vi "CAN_Send Diag Message.vi"(0 "Write Session in":refnum<k21>, 1 "Read Session in":refnum<k21>, 2 "Parttype ref":refnum<vi>, 3 "ODX File Path":path=path "C:/LegacyApp/DB_0CA_7100_4M0_0004_73710BVW3710/DB_0CA_7100_4M0_0004_73710BVW3710/DB_0CA_7100_4M0_0004_73710BVW3710.odx", 4 "Tx Msg":u8[](array[numeric])=[2, 26, 156, 255, 255, 255, 255, 255] format="%02x", 5 "error in (no error)":errorcluster, 6 "Enum":T2=enum."Get Calibration Status", 7 "Download CAL Progress":refnum<vi>, 10 "Postion":u16=3, 11 "Download CAL Time":refnum<vi>, 12 "Autotest":bool, 14 "ECU Info in":T1, 17 "Tester":refnum<k21>) -> (13 "Response Good?":bool, 15 "ECU Info":T1, 16 "pass?":bool, 18 "TxRx Data":string[][](array[string]), 19 "error out":errorcluster)   [LabVIEW 2018]
uses:
  Diagnostic Message.ctl
  typedefs/parttype.ctl
  <vilib>/xnet/xnet.llb/XNET Frame CAN.ctl
  <vilib>/xnet/xnet.llb/XNET Frame Type CAN.ctl
  CAN Communication VI's/Typedefs/Select Session.ctl
  typedefs/All Motions.ctl
  <vilib>/xnet/xnet.llb/XNET Write (Frame CAN).vi
  <vilib>/xnet/xnet.llb/XNET Read (Frame CAN).vi
panel:
  out "Error String Out 2":string
  out "pass?_FBL":bool
  out "Rx Message":u8[](array[numeric]) format="%02x"
  out "Error String Out":string
  in  "Tx Arbitration Id":u32=402391172 format="%.0x"
  out "Part Number":string
  out "Vehicle Type":string
  out "SW level":string
  out "Calibrated":bool
  out "HW level":string
  out "CAL level":string
  out "Boot level":string
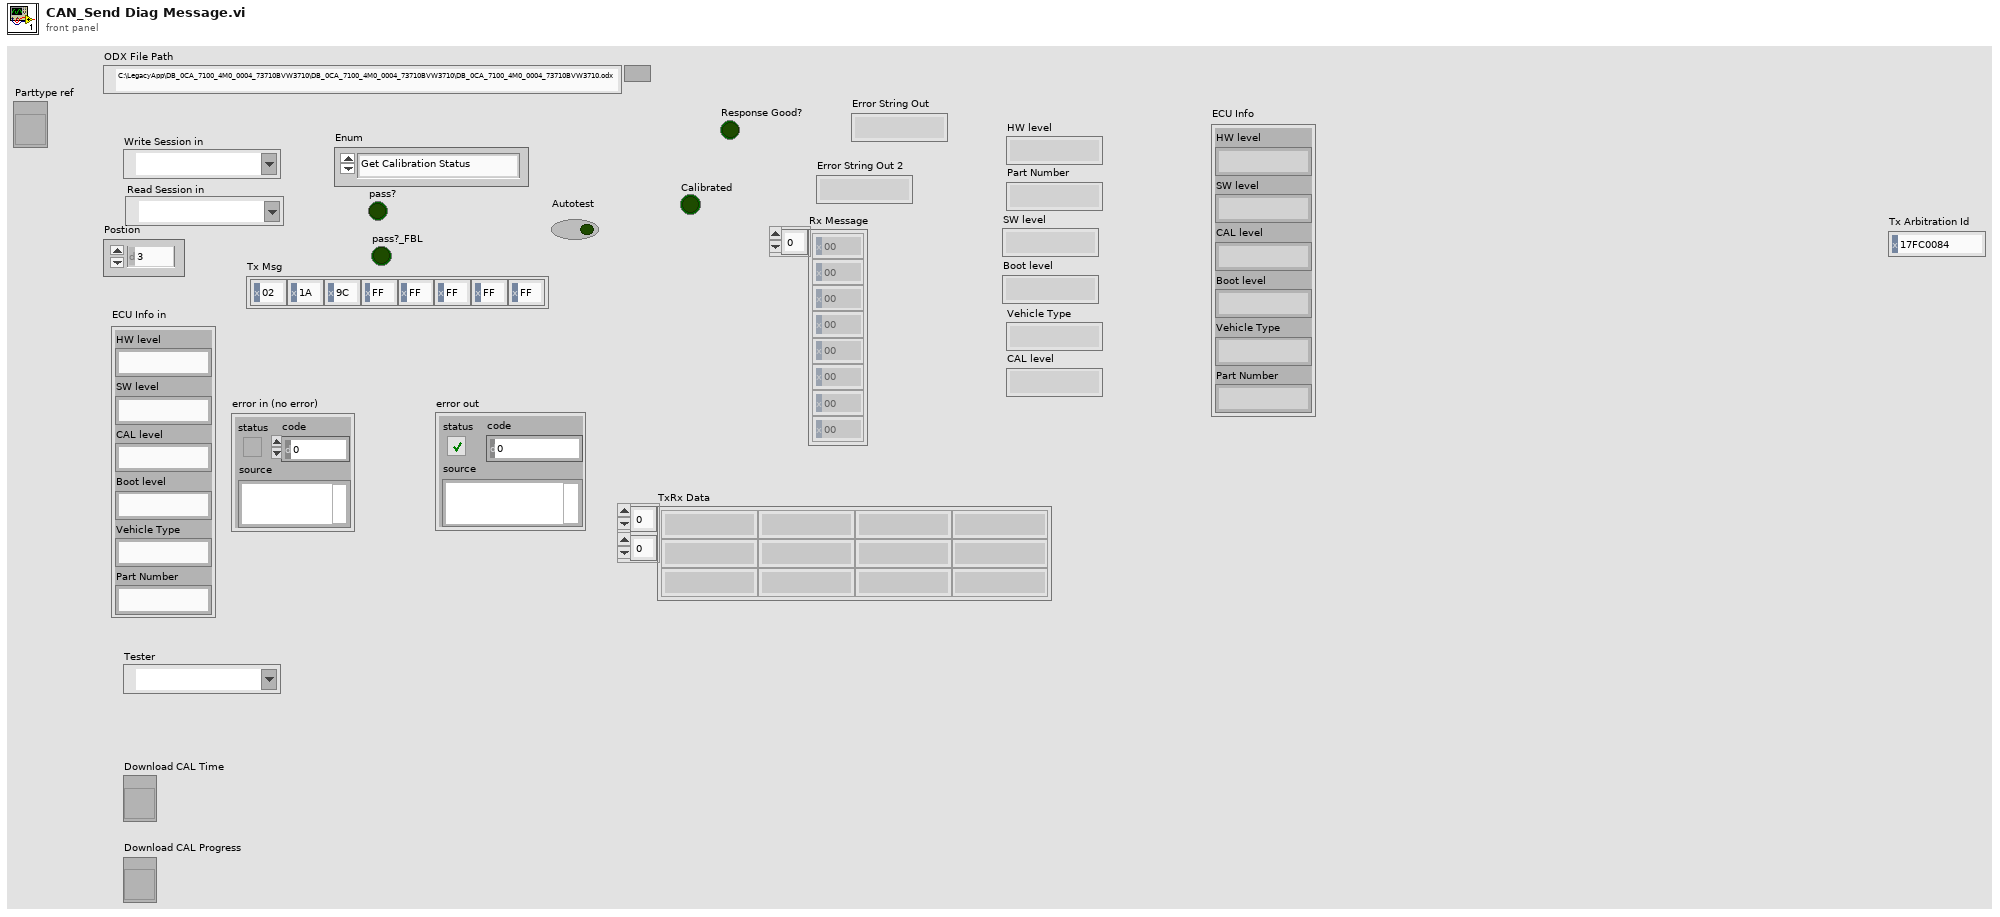
[diagram p1: front panel]
types:
  T1 = cluster{"HW level":string, "SW level":string, "CAL level":string, "Boot level":string, "Vehicle Type":string, "Part Number":string}
  T2 = typedef "Diagnostic Message.ctl" = enum16{"User Select", "Get User Multi-Frame", "Diag Session Prog", "Diag Session Ext", "Diag Session EOL", "Diag Session Default", "Diag Session Dev", "Read Active Session", "Read HW", "Read SW", "Read Part Number", "Learn Start Glass", "Learn Start Rollo", "Get Calibration Status", "Read SW CAL Boot", "Go to Position", "Get Parametric Mode Status", "Enable Parametric Mode", "Disable Parametric Mode", "Enable Production Mode", "Disable Production Mode", "Reset ECU", "Go to Slide Close", "Go to Slide Open", "Go to Vent Open", "Rollo Open", "Rollo Close", "Write Vehicle Type", "Read Vehicle Type", "Clear DTC", "Check Teach DTC", "Write Shop Code", "Download CAL", "Finish Flash", "Delete RP RF", "Download FBL"}
  T3 = typedef "XNET Frame CAN.ctl" = cluster{"timestamp":timestamp, "payload":u8[], "identifier":u32, "type":T4, "extended?":bool, "echo?":bool}
  T4 = typedef "XNET Frame Type CAN.ctl" = u8
  T5 = typedef "Select Session.ctl" = enum16{"DefaultSession", "Development", "Extended", "EOL", "Programming"}
  T6 = typedef "All Motions.ctl" = enum16{"Idle", "Glass Teach", "Glass Slide Open", "Glass Slide Open 2", "Glass Slide Close", "Glass Slide Close 2", "Glass Vent Open", "Glass Vent Close", "Sunshade Teach", "Sunshade Teach 2", "Sunshade Open", "Sunshade Open 2", "Sunshade Close", "Sunshade Close 2", "Glass Slide Open Sunshade Open", "Glass Slide Open 2 Sunshade Open", "Glass Slide Open Sunshade Close", "Glass Slide Open 2 Sunshade Close", "Glass Slide Close Sunshade Open", "Glass Slide Close 2 Sunshade Open", "Glass Slide Close Sunshade Close", "Glass Slide Close 2 Sunshade Close", "Glass Vent Open Sunshade Open", "Glass Vent Open Sunshade Close", "Glass Vent Close Sunshade Open", "Glass Vent Close Sunshade Close", "Express Glass Slide Open", "Express Glass Slide Open 2", "Express Glass Slide Close", "Express Glass Slide Close 2", "Express Glass Vent Open", "Express Glass Vent Close", "Express Sunshade Open", "Express Sunshade Close", "Express Sunshade Open 2", "Express Sunshade Close 2", "Express Glass Slide Open Sunshade Open", "Express Glass Slide Open 2 Sunshade Open", "Express Glass Slide Open Sunshade Close", "Express Glass Slide Open 2 Sunshade Close", "Express Glass Slide Close Sunshade Open", "Express Glass Slide Close 2 Sunshade Open", "Express Glass Slide Close Sunshade Close", "Express Glass Slide Close 2 Sunshade Close", "Express Glass Vent Open Sunshade Open", "Express Glass Vent Open Sunshade Close", "Express Glass Vent Close Sunshade Open", "Express Glass Vent Close Sunshade Close", "Goto Position Glass", "Goto Position Sunshade"}
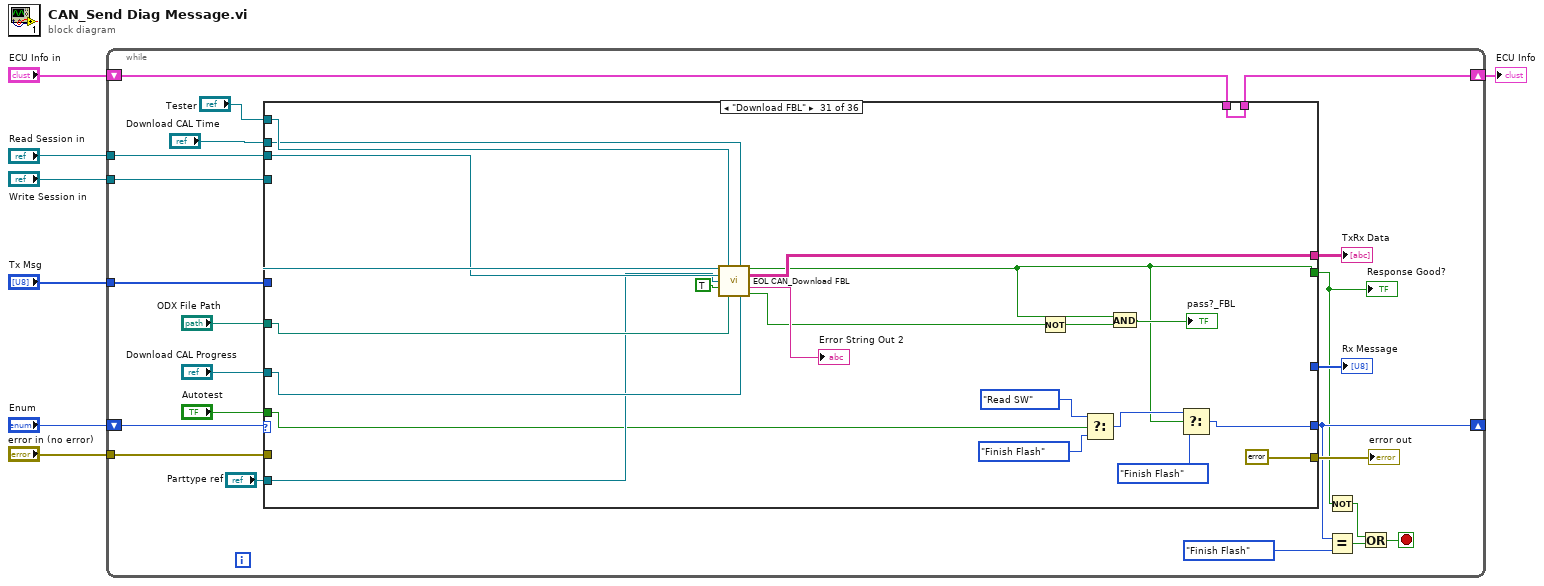
[diagram p0: block diagram]
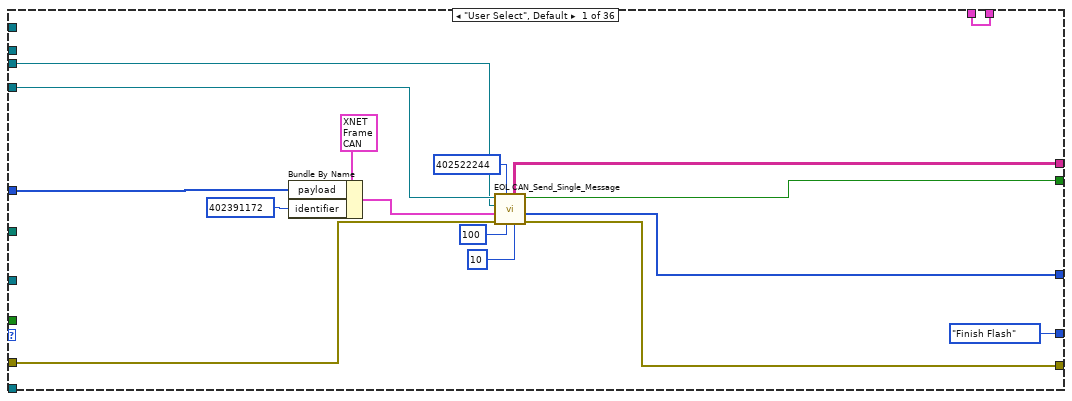
[diagram p2: hidden frame]
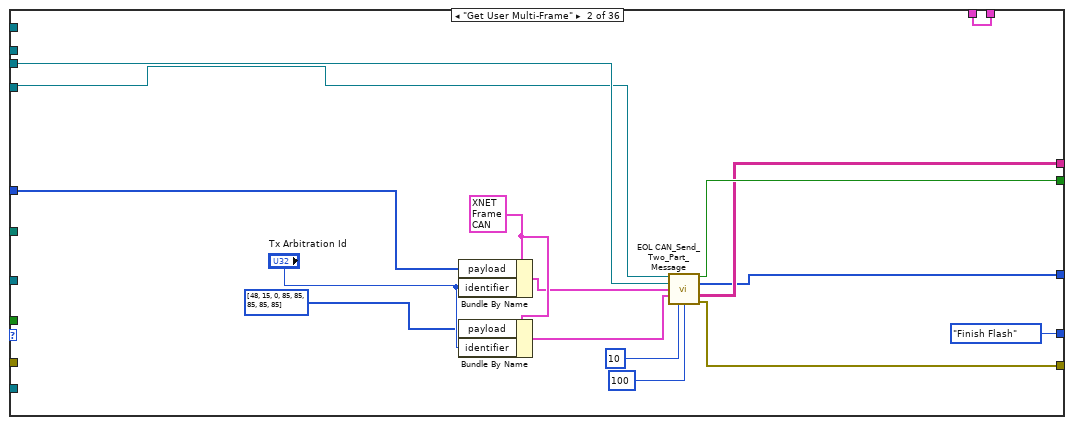
[diagram p3: hidden frame]
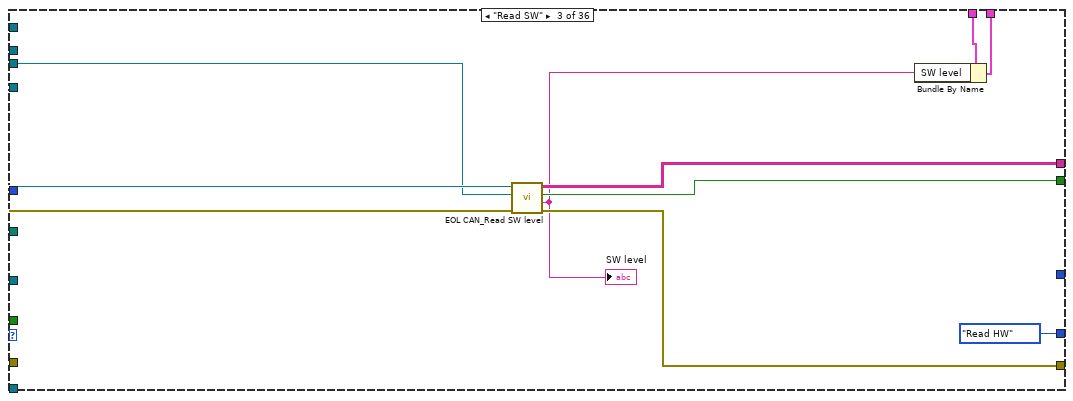
[diagram p4: hidden frame]
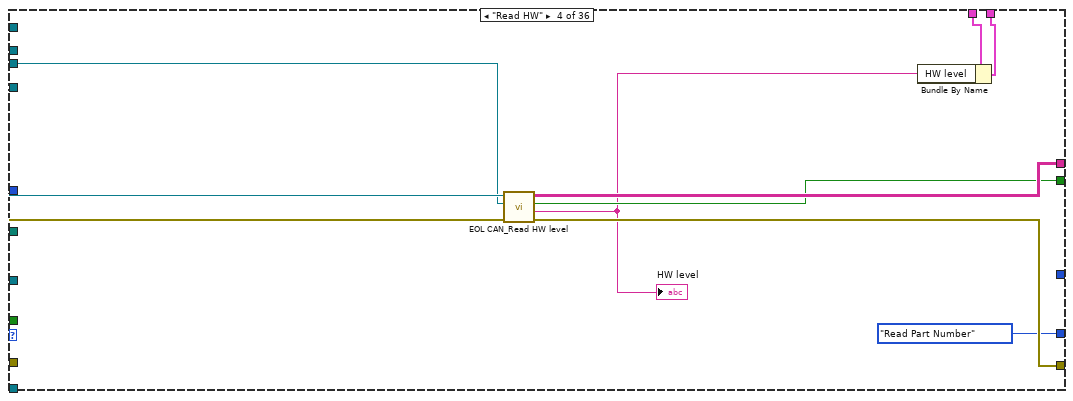
[diagram p5: hidden frame]
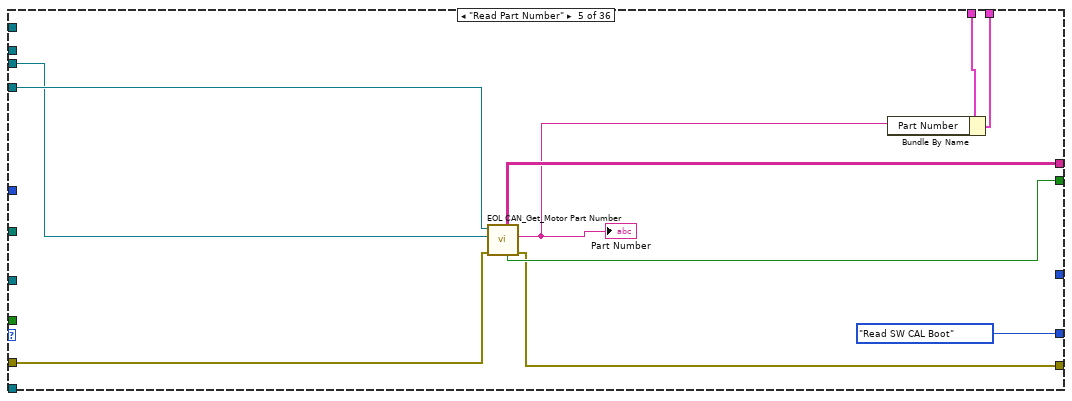
[diagram p6: hidden frame]
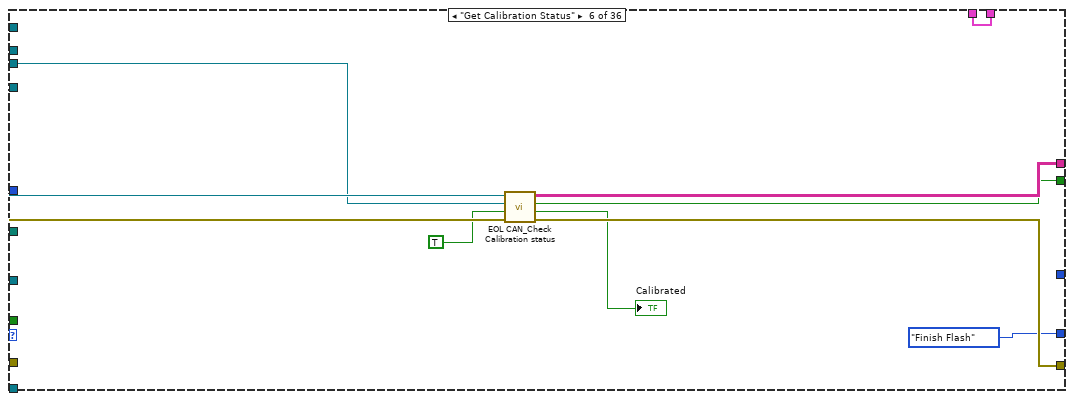
[diagram p7: hidden frame]
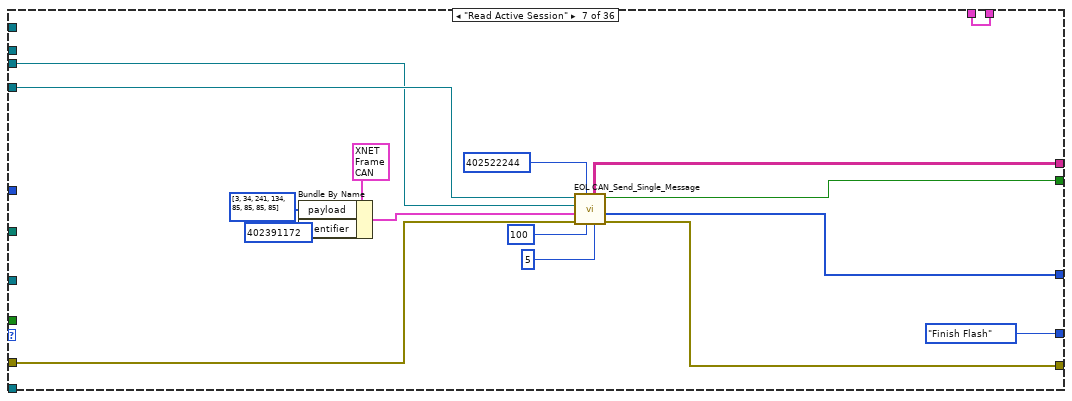
[diagram p8: hidden frame]
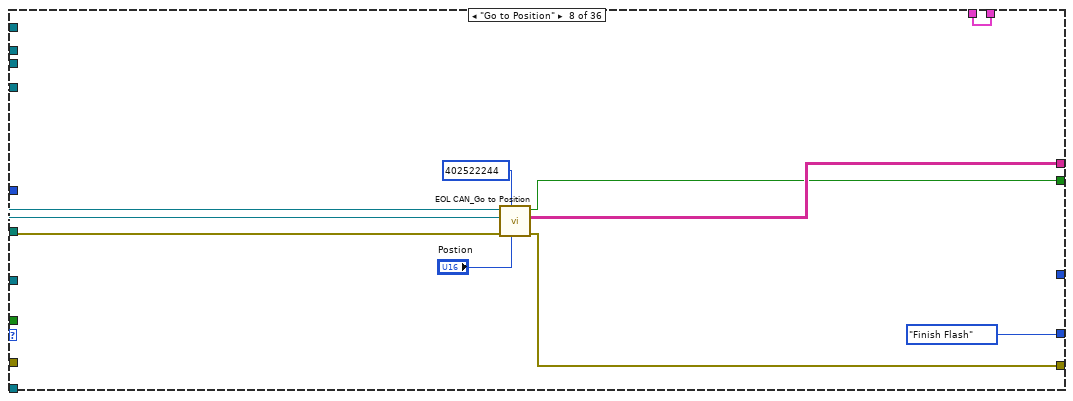
[diagram p9: hidden frame]
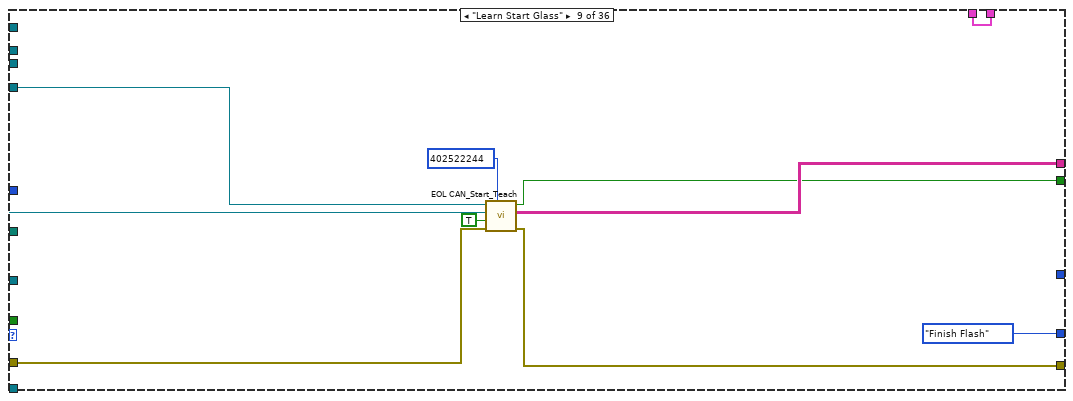
[diagram p10: hidden frame]
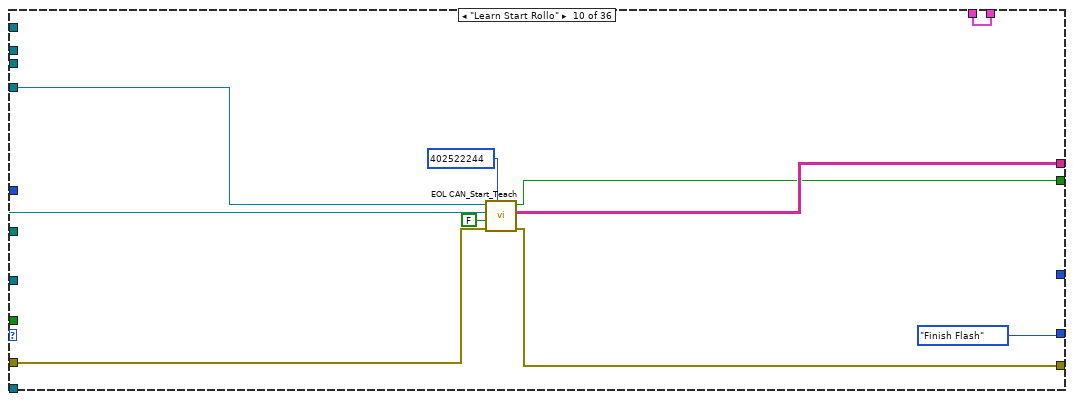
[diagram p11: hidden frame]
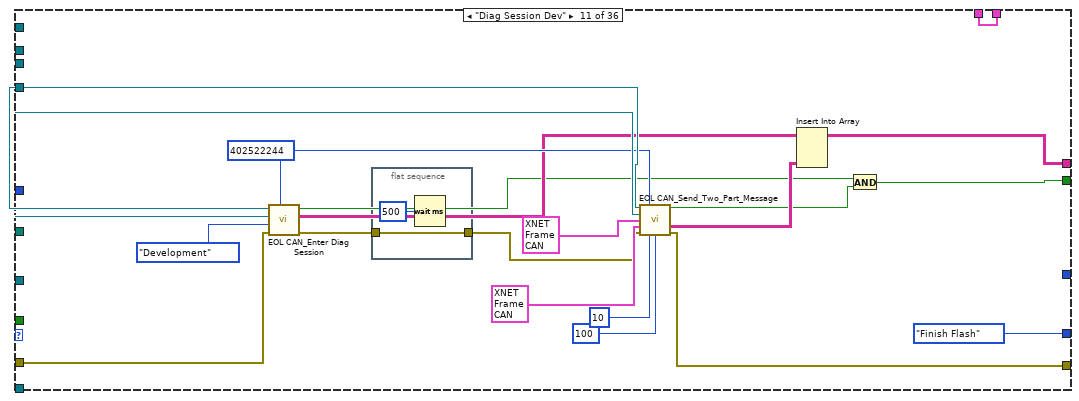
[diagram p12: hidden frame]
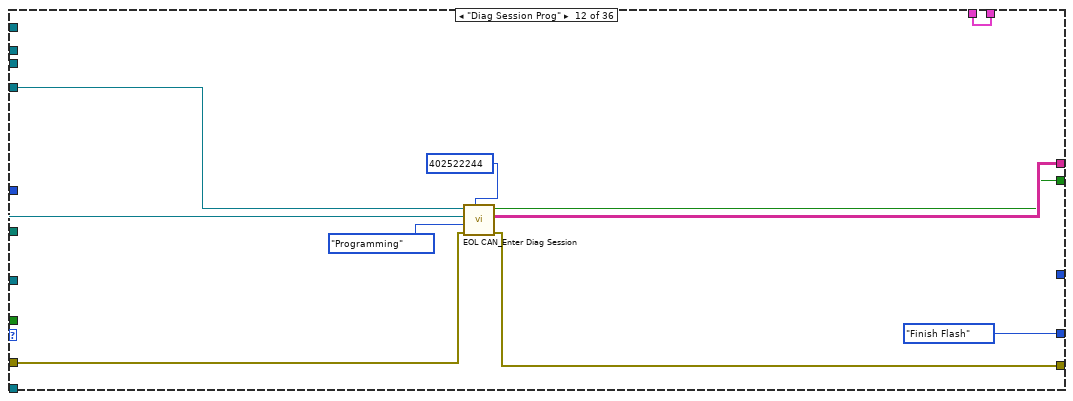
[diagram p13: hidden frame]
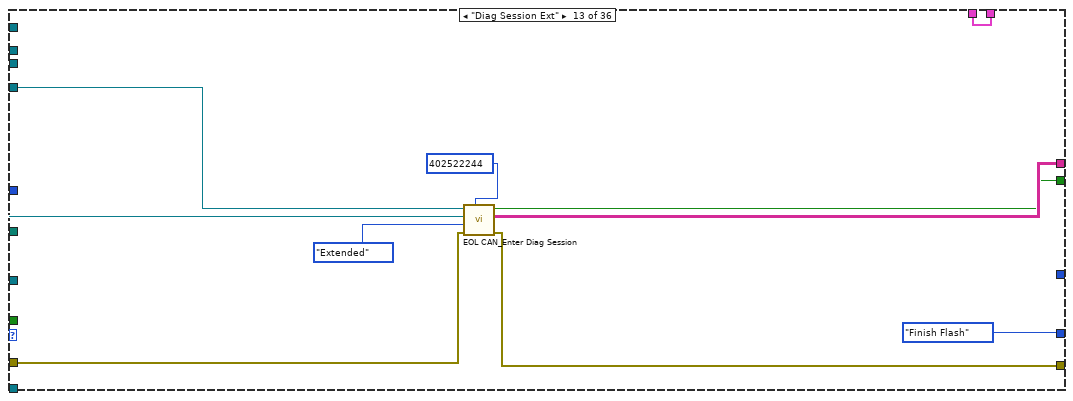
[diagram p14: hidden frame]
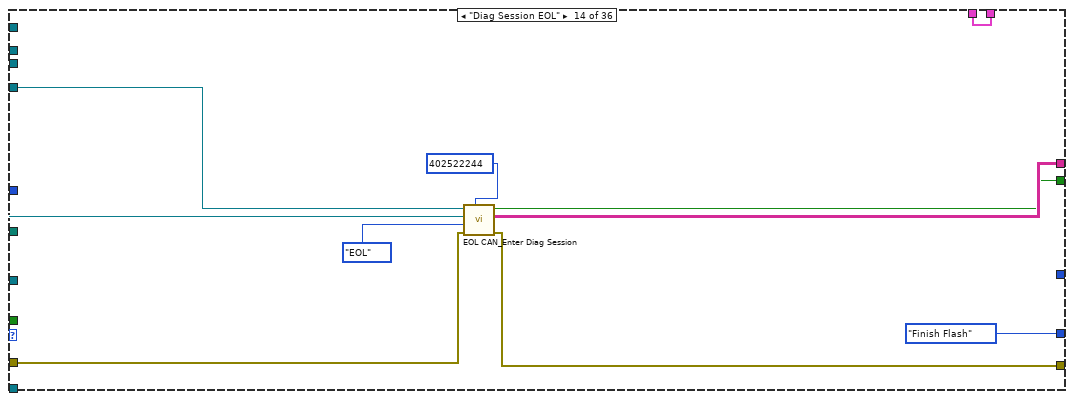
[diagram p15: hidden frame]
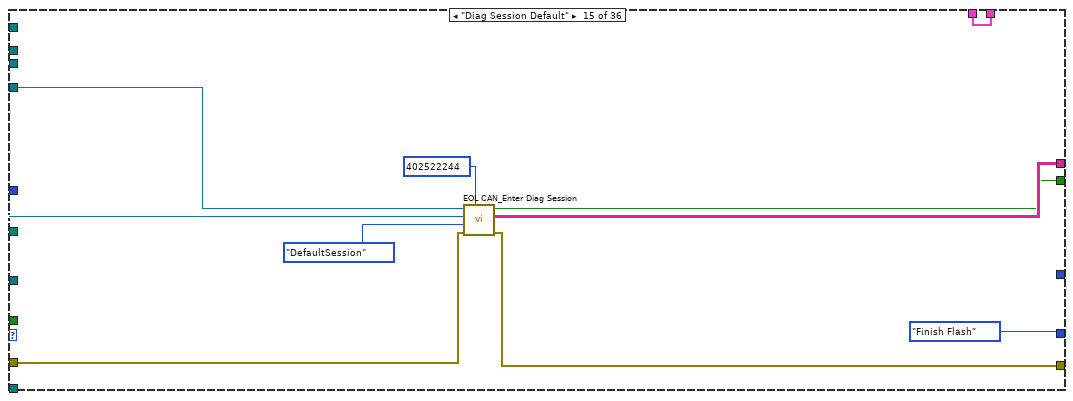
[diagram p16: hidden frame]
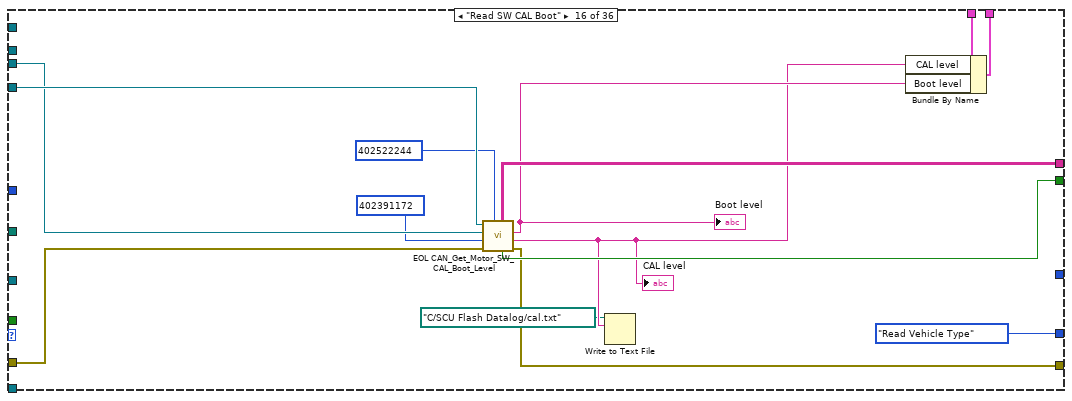
[diagram p17: hidden frame]
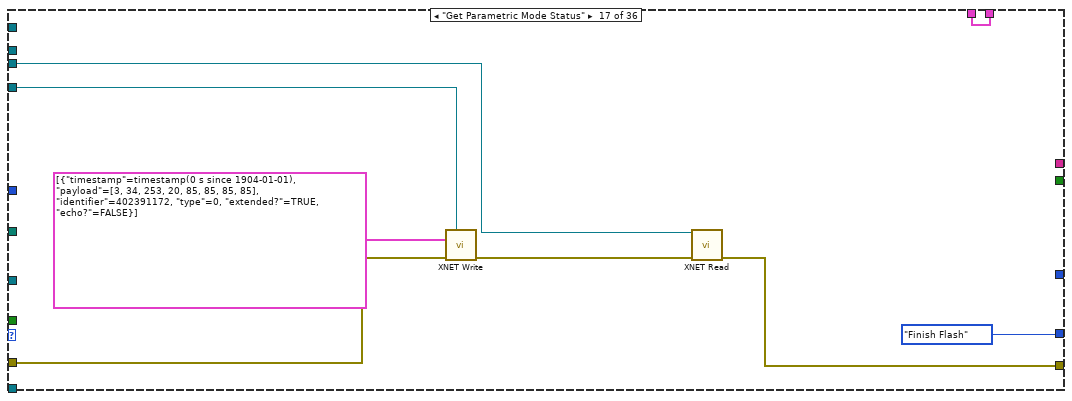
[diagram p18: hidden frame]
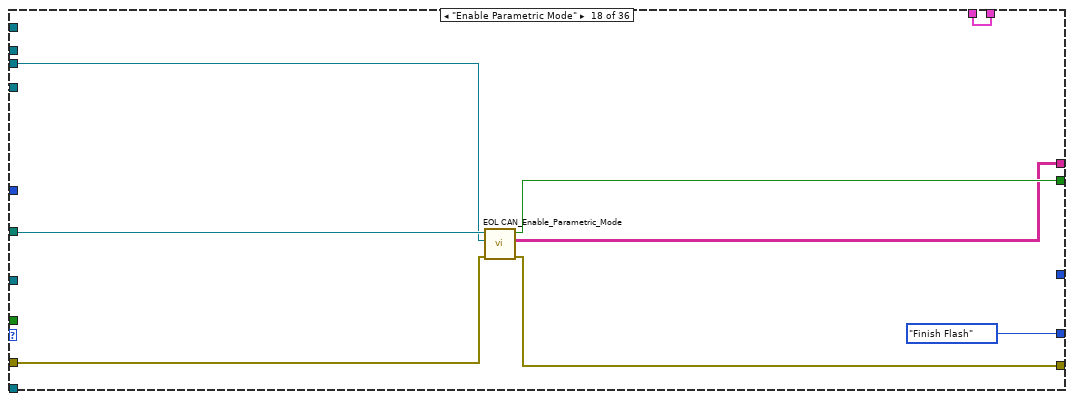
[diagram p19: hidden frame]
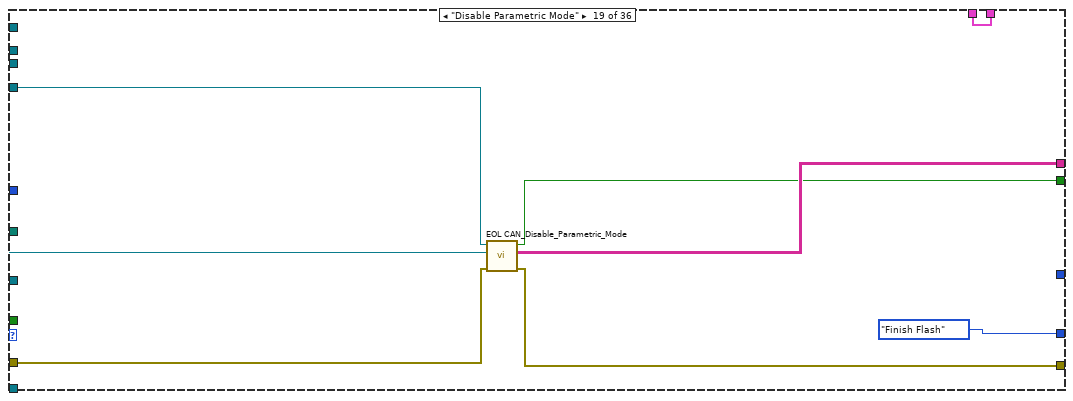
[diagram p20: hidden frame]
diagram:
  n1 = while {
    tunnel: "error in (no error)" -> [w29]
    tunnel: "Read Session in" -> [w27]
    tunnel: "Write Session in" -> [w26]
    shift-right: [w23] -> w3
    shift-left: "ECU Info in" -> [w22]
    tunnel: "Tx Msg" -> [w21]
    shift-right: [w16] -> _
    shift-left: "Enum" -> [w25]
    stop <- w19 stop-if-true
    n2 = case shown="\"Download FBL\"" w25 {
      tunnel: w27 -> [w44 w53 w66 w76 w89 w100 w116 w124 w135 w145 w163 w173 w183 w193 w203 w221 w229 w237 w242 w253 w261 w270 w280 w290 w300 w310 w320 w324 w332 w357 w379 w393 w400 w410 _ w439]
      tunnel: w26 -> [w45 w52 w67 w77 w90 w101 w117 w125 w136 w146 w165 w174 w184 w194 w204 w222 w231 w238 w243 w254 w262 w271 w281 w291 w301 w311 w321 w325 w333 w358 w380 w392 w401 w412 _ w440]
      tunnel: w29 -> [w43 _ w71 w81 w91 w99 w115 w127 w137 w147 w167 w179 w189 w199 w209 w223 w230 w239 w247 w255 w263 w272 w282 w292 w302 w312 w322 _ _ _ _ w394 w402 w411 w430 w434]
      tunnel: [w42 w48 w70 w80 w86 w98 w114 w126 w133 w143 w164 w178 w188 w198 w208 w216 w226 w234 w246 w250 w258 w266 w276 w286 w296 w306 w316 w328 w336 errorcluster {"status"=FALSE, "code"=0, "source"=""} ("error IO") errorcluster {"status"=FALSE, "code"=0, "source"=""} ("error IO") w387 w399 w409 w430 w436] -> w28
      tunnel: [w41 w49 w69 w79 w88 w97 w113 w122 w132 w142 w157 w177 w187 w197 w207 w218 _ w235 w245 w251 w259 w268 w277 w287 w297 w307 w317 w329 w337 w355 w377 w389 w397 _ _ w438] -> w24
      tunnel: [w40 w50 w68 w78 w87 w94 w112 w121 w131 w141 w154 w176 w186 w196 w206 w217 _ w236 w244 w252 w260 w267 w278 w288 w298 w308 w318 w327 w335 w347 w361 w388 w398 _ _ w437] -> w15
      tunnel: [w39 w47 _ _ _ _ w109 _ _ _ _ _ _ _ _ _ _ _ _ _ _ _ _ _ _ _ _ w326 w334 _ _ _ _ _ _ _] -> w20
      tunnel: [w32 w61 w64 w73 w84 w93 w103 w119 w130 w140 w149 w171 w181 w191 w201 w214 w225 w233 w241 w249 w257 w265 w274 w284 w294 w304 w314 w330 w338 w360 w382 w385 w396 w404 w431 w441] -> w23
      tunnel: w22 -> [w32 w61 w65 w74 w83 w93 w103 w119 w130 w140 w149 w171 w181 w191 w201 w215 w225 w233 w241 w249 w257 w265 w274 w284 w294 w304 w314 w330 w338 w360 w382 w386 w396 w404 w431 w441]
      tunnel: w21 -> [w31 w51 _ _ _ _ _ _ _ _ _ _ _ _ _ _ _ _ _ _ _ _ _ _ _ _ _ _ _ _ _ _ _ _ _ _]
      tunnel: [Diagnostic_Message."Finish Flash" ("Enum") Diagnostic_Message."Finish Flash" ("Enum") Diagnostic_Message."Read HW" ("Enum") Diagnostic_Message."Read Part Number" ("Enum") Diagnostic_Message."Read SW CAL Boot" ("Enum") Diagnostic_Message."Finish Flash" ("Enum") Diagnostic_Message."Finish Flash" ("Enum") Diagnostic_Message."Finish Flash" ("Enum") Diagnostic_Message."Finish Flash" ("Enum") Diagnostic_Message."Finish Flash" ("Enum") Diagnostic_Message."Finish Flash" ("Enum") Diagnostic_Message."Finish Flash" ("Enum") Diagnostic_Message."Finish Flash" ("Enum") Diagnostic_Message."Finish Flash" ("Enum") Diagnostic_Message."Finish Flash" ("Enum") Diagnostic_Message."Read Vehicle Type" ("Enum") Diagnostic_Message."Finish Flash" ("Enum") Diagnostic_Message."Finish Flash" ("Enum") Diagnostic_Message."Finish Flash" ("Enum") Diagnostic_Message."Delete RP RF" ("Enum") Diagnostic_Message."Finish Flash" ("Enum") Diagnostic_Message."Finish Flash" ("Enum") Diagnostic_Message."Finish Flash" ("Enum") Diagnostic_Message."Finish Flash" ("Enum") Diagnostic_Message."Finish Flash" ("Enum") Diagnostic_Message."Finish Flash" ("Enum") Diagnostic_Message."Finish Flash" ("Enum") Diagnostic_Message."Finish Flash" ("Enum") Diagnostic_Message."Finish Flash" ("Enum") w350 w372 Diagnostic_Message."Enable Production Mode" ("Enum") Diagnostic_Message."Finish Flash" ("Enum") Diagnostic_Message."Finish Flash" ("Enum") Diagnostic_Message."Finish Flash" ("Enum") Diagnostic_Message."Finish Flash" ("Enum")] -> w16
      tunnel: "Tester" -> [_ _ _ _ _ _ _ _ _ _ _ _ _ _ _ _ _ _ _ _ _ _ _ _ _ _ _ _ _ w344 w367 _ _ _ _ _]
      tunnel: "Download CAL Time" -> [_ _ _ _ _ _ _ _ _ _ _ _ _ _ _ _ _ _ _ _ _ _ _ _ _ _ _ _ _ w343 w366 _ _ _ _ _]
      tunnel: "ODX File Path" -> [_ _ _ _ _ _ _ _ _ _ _ _ _ _ _ _ _ _ _ _ _ _ _ _ _ _ _ _ _ w342 w365 _ _ _ _ _]
      tunnel: "Download CAL Progress" -> [_ _ _ _ _ _ _ _ _ _ _ _ _ _ _ _ _ _ _ _ _ _ _ _ _ _ _ _ _ w341 w364 _ _ _ _ _]
      tunnel: "Parttype ref" -> [_ _ _ _ _ _ _ _ _ _ _ _ _ _ _ _ _ _ _ _ _ _ _ _ _ _ _ _ _ w340 w363 _ _ _ _ _]
      tunnel: "Autotest" -> [_ _ _ _ _ _ _ _ _ _ _ _ _ _ _ _ _ _ _ _ _ _ _ _ _ _ _ _ _ w339 w362 _ _ _ _ _]
      frame "User Select", Default {
        n3 = Bundle By Name(cluster=T3 {"timestamp"=timestamp(0 s since 1904-01-01), "payload"=[2, 39, 3, 85, 85, 85, 85, 85], "identifier"=402391172, "type"=0, "extended?"=TRUE, "echo?"=FALSE} ("Tx CAN frame"), "payload"=w31, "identifier"=u32 402391172) -> (w37:T3)
        n4 = call "EOL CAN_Send_Single_Message.vi"("Retries"=10, "Msg Wait Time"=u32 100, "Rx Arbitration Id"=u32 402522244, "Error in"=w43, "Tx CAN frame"=w37, "Read Session in"=w44, "Write Session in"=w45) -> ("Error out"=w42:errorcluster, "Rx Message"=w39:u8[], "Response Good?"=w40:bool, "TxRx Data"=w41:string[][])  [unwired: 1 out]
      }
      frame "Get User Multi-Frame" {
        w55 = T3 {"timestamp"=timestamp(0 s since 1904-01-01), "payload"=[2, 39, 3, 85, 85, 85, 85, 85], "identifier"=402391172, "type"=0, "extended?"=TRUE, "echo?"=FALSE} ("Tx CAN frame 1")
        n5 = Bundle By Name(cluster=w55, "payload"=w51, "identifier"="Tx Arbitration Id") -> (w54:T3)
        n6 = Bundle By Name(cluster=w55, "payload"=u8[] [48, 15, 0, 85, 85, 85, 85, 85] ("Transmit Data"), "identifier"="Tx Arbitration Id") -> (w56:T3)
        n7 = call "EOL CAN_Send_Two_Part_Message.vi"("Write Session in"=w52, "Read Session in"=w53, "Tx CAN frame 1"=w54, "Tx CAN frame 2"=w56, "Retries"=10, "Msg Wait Time"=u32 100) -> ("Response Good?"=w50:bool, "Rx Data"=w47:u8[], "TxRx Data"=w49:string[][], "error out"=w48:errorcluster)  [unwired: 6 in]
      }
      frame "Read SW" {
        n8 = call "EOL CAN_Read SW level.vi"("error in (no error)"=w71, "Read Session in"=w66, "Write Session in"=w67) -> ("error out"=w70:errorcluster, "SW level"=w63:string, "Response Good?"=w68:bool, "TxRx Data"=w69:string[][])  [unwired: 5 in]
        "SW level" <- w63
        n9 = Bundle By Name(cluster=w65, "SW level"=w63) -> (w64:T1)
      }
      frame "Read HW" {
        n10 = call "EOL CAN_Read HW level.vi"("error in (no error)"=w81, "Read Session in"=w76, "Write Session in"=w77) -> ("error out"=w80:errorcluster, "HW level"=w75:string, "Response Good?"=w78:bool, "TxRx Data"=w79:string[][])  [unwired: 5 in]
        "HW level" <- w75
        n11 = Bundle By Name(cluster=w74, "HW level"=w75) -> (w73:T1)
      }
      frame "Read Part Number" {
        n12 = call "EOL CAN_Get_Motor Part Number.vi"("error in (no error)"=w91, "Read Session in"=w89, "Write Session in"=w90) -> ("error out"=w86:errorcluster, "Part Number"=w85:string, "Response Good?"=w87:bool, "TxRx Data"=w88:string[][])  [unwired: 5 in]
        "Part Number" <- w85
        n13 = Bundle By Name(cluster=w83, "Part Number"=w85) -> (w84:T1)
      }
      frame "Get Calibration Status" {
        n14 = call "EOL CAN_Check Calibration status.vi"("error in (no error)"=w99, "Glass?"=TRUE, "Read Session in"=w100, "Write Session in"=w101) -> ("error out"=w98:errorcluster, "Calibrated"=→"Calibrated":bool, "Response Good?"=w94:bool, "TxRx Data"=w97:string[][])  [unwired: 4 in]
      }
      frame "Read Active Session" {
        n15 = Bundle By Name(cluster=T3 {"timestamp"=timestamp(0 s since 1904-01-01), "payload"=[2, 39, 3, 85, 85, 85, 85, 85], "identifier"=402391172, "type"=0, "extended?"=TRUE, "echo?"=FALSE} ("Tx CAN frame"), "payload"=u8[] [3, 34, 241, 134, 85, 85, 85, 85], "identifier"=u32 402391172) -> (w106:T3)
        n16 = call "EOL CAN_Send_Single_Message.vi"("Retries"=5, "Msg Wait Time"=u32 100, "Rx Arbitration Id"=u32 402522244, "Error in"=w115, "Tx CAN frame"=w106, "Read Session in"=w116, "Write Session in"=w117) -> ("Error out"=w114:errorcluster, "Rx Message"=w109:u8[], "Response Good?"=w112:bool, "TxRx Data"=w113:string[][])  [unwired: 1 out]
      }
      frame "Go to Position" {
        n17 = call "EOL CAN_Go to Position.vi"("Postion"="Postion", "Rx Arbitration Id"=u32 402522244, "Error in"=w127, "Read Session in"=w124, "Write Session in"=w125) -> ("Error out"=w126:errorcluster, "TxRx Data"=w122:string[][], "Response Good?"=w121:bool)  [unwired: 4 in]
      }
      frame "Learn Start Glass" {
        n18 = call "EOL CAN_Start_Teach.vi"("Rx Arbitration Id"=u32 402522244, "Error in"=w137, "Glass?"=TRUE, "Read Session in"=w135, "Write Session in"=w136) -> ("Error out"=w133:errorcluster, "TxRx Data"=w132:string[][], "Response Good?"=w131:bool)  [unwired: 4 in]
      }
      frame "Learn Start Rollo" {
        n19 = call "EOL CAN_Start_Teach.vi"("Rx Arbitration Id"=u32 402522244, "Error in"=w147, "Glass?"=FALSE, "Read Session in"=w145, "Write Session in"=w146) -> ("Error out"=w143:errorcluster, "TxRx Data"=w142:string[][], "Response Good?"=w141:bool)  [unwired: 4 in]
      }
      frame "Diag Session Dev" {
        w162 = u32 402522244 ("Rx Arbitration Id")
        n20 = call "EOL CAN_Enter Diag Session.vi"("Rx Arbitration Id"=w162, "Error in"=w167, "Session"=Select_Session."Development", "Read Session in"=w163, "Write Session in"=w165) -> ("Error out"=w153:errorcluster, "TxRx Data"=w159:string[][], "Response Good?"=w155:bool)  [unwired: 4 in]
        n21 = flat-sequence {
          tunnel: w153 -> [w168]
          tunnel: [w168] -> w152
          frame #0 {
            n22 = Wait (ms)(milliseconds to wait=u32 500) -> ()  [unwired: 1 out]
          }
        }
        n23 = call "EOL CAN_Send_Two_Part_Message.vi"("Write Session in"=w165, "Rx Arbitration Id"=w162, "Read Session in"=w163, "Tx CAN frame 1"=T3 {"timestamp"=timestamp(0 s since 1904-01-01), "payload"=[3, 34, 254, 253, 85, 85, 85, 85], "identifier"=402391172, "type"=8, "extended?"=TRUE, "echo?"=FALSE}, "Tx CAN frame 2"=T3 {"timestamp"=timestamp(0 s since 1904-01-01), "payload"=[48, 15, 0, 85, 85, 85, 85, 85], "identifier"=402391172, "type"=8, "extended?"=TRUE, "echo?"=FALSE}, "error in (no error)"=w152, "Retries"=10, "Msg Wait Time"=u32 100) -> ("Response Good?"=w156:bool, "TxRx Data"=w158:string[][], "error out"=w164:errorcluster)  [unwired: 4 in, 1 out]
        n24 = Insert Into Array(array=w159, new element=w158) -> (w157:string[][])  [unwired: 2 in]
        n25 = And(x=w155, y=w156) -> (x .and. y?=w154:bool)
      }
      frame "Diag Session Prog" {
        n26 = call "EOL CAN_Enter Diag Session.vi"("Rx Arbitration Id"=u32 402522244, "Error in"=w179, "Session"=Select_Session."Programming", "Read Session in"=w173, "Write Session in"=w174) -> ("Error out"=w178:errorcluster, "TxRx Data"=w177:string[][], "Response Good?"=w176:bool)  [unwired: 4 in]
      }
      frame "Diag Session Ext" {
        n27 = call "EOL CAN_Enter Diag Session.vi"("Rx Arbitration Id"=u32 402522244, "Error in"=w189, "Session"=Select_Session."Extended", "Read Session in"=w183, "Write Session in"=w184) -> ("Error out"=w188:errorcluster, "TxRx Data"=w187:string[][], "Response Good?"=w186:bool)  [unwired: 4 in]
      }
      frame "Diag Session EOL" {
        n28 = call "EOL CAN_Enter Diag Session.vi"("Rx Arbitration Id"=u32 402522244, "Error in"=w199, "Session"=Select_Session."EOL", "Read Session in"=w193, "Write Session in"=w194) -> ("Error out"=w198:errorcluster, "TxRx Data"=w197:string[][], "Response Good?"=w196:bool)  [unwired: 4 in]
      }
      frame "Diag Session Default" {
        n29 = call "EOL CAN_Enter Diag Session.vi"("Rx Arbitration Id"=u32 402522244, "Error in"=w209, "Session"=Select_Session."DefaultSession", "Read Session in"=w203, "Write Session in"=w204) -> ("Error out"=w208:errorcluster, "TxRx Data"=w207:string[][], "Response Good?"=w206:bool)  [unwired: 4 in]
      }
      frame "Read SW CAL Boot" {
        n30 = call "EOL CAN_Get_Motor_SW_CAL_Boot_Level.vi"("Rx Arbitration Id"=u32 402522244, "error in (no error)"=w223, "Tx Arbitration Id"=u32 402391172 ("identifier"), "Read Session in"=w221, "Write Session in"=w222) -> ("error out"=w216:errorcluster, "CAL level"=w211:string, "Boot level"=w213:string, "Response Good?"=w217:bool, "TxRx Data"=w218:string[][])  [unwired: 1 in, 1 out]
        "Boot level" <- w213
        "CAL level" <- w211
        n31 = Write to Text File(file (use dialog)=path "C:/SCU Flash Datalog/cal.txt", text=w211) -> ()  [unwired: 2 in, 3 out]
        n32 = Bundle By Name(cluster=w215, "CAL level"=w211, "Boot level"=w213) -> (w214:T1)
      }
      frame "Get Parametric Mode Status" {
        n33 = call-poly <vilib>:"XNET Write.vi"("session in"=w231, "data"=T3[] [{"timestamp"=timestamp(0 s since 1904-01-01), "payload"=[3, 34, 253, 20, 85, 85, 85, 85], "identifier"=402391172, "type"=0, "extended?"=TRUE, "echo?"=FALSE}] ("Frame to Send 2"), "error in (no error)"=w230) -> ("error out"=w227:errorcluster)  [unwired: 11 in, 1 out]
        n34 = call-poly <vilib>:"XNET Read.vi"("session in"=w229, "error in (no error)"=w227) -> ("error out"=w226:errorcluster)  [unwired: 10 in, 3 out]
      }
      frame "Enable Parametric Mode" {
        n35 = call "EOL CAN_Enable_Parametric_Mode.vi"("Error in"=w239, "Read Session in"=w237, "Write Session in"=w238) -> ("Error out"=w234:errorcluster, "debug log"=w235:string[][], "Response Good?"=w236:bool)  [unwired: 6 in]
      }
      frame "Disable Parametric Mode" {
        n36 = call "EOL CAN_Disable_Parametric_Mode.vi"("Error in"=w247, "Read Session in"=w242, "Write Session in"=w243) -> ("Error out"=w246:errorcluster, "debug log"=w245:string[][], "Response Good?"=w244:bool)  [unwired: 6 in]
      }
      frame "Enable Production Mode" {
        n37 = call "EOL CAN_Enable_Production_Mode.vi"("Error in"=w255, "Read Session in"=w253, "Write Session in"=w254) -> ("Error out"=w250:errorcluster, "debug log"=w251:string[][], "Response Good?"=w252:bool)  [unwired: 6 in]
      }
      frame "Disable Production Mode" {
        n38 = call "EOL CAN_Disable_Production_Mode.vi"("Error in"=w263, "Read Session in"=w261, "Write Session in"=w262) -> ("Error out"=w258:errorcluster, "debug log"=w259:string[][], "Response Good?"=w260:bool)  [unwired: 6 in]
      }
      frame "Reset ECU" {
        n39 = call "EOL CAN_Reset ECU.vi"("Rx Arbitration Id"=u32 402522244, "Error in"=w272, "Read Session in"=w270, "Write Session in"=w271) -> ("Error out"=w266:errorcluster, "Response Good?"=w267:bool, "TxRx Data"=w268:string[][])  [unwired: 5 in]
      }
      frame "Go to Slide Close" {
        n40 = call "EOL CAN_Target Motion.vi"("Rx Arbitration Id"=u32 402522244, "Error in"=w282, "All Motions"=All_Motions."Glass Slide Close", "Read Session in"=w280, "Write Session in"=w281) -> ("Error out"=w276:errorcluster, "TxRx Data"=w277:string[][], "Response Good?"=w278:bool)  [unwired: 4 in]
      }
      frame "Go to Slide Open" {
        n41 = call "EOL CAN_Target Motion.vi"("Rx Arbitration Id"=u32 402522244, "Error in"=w292, "All Motions"=All_Motions."Glass Slide Open", "Read Session in"=w290, "Write Session in"=w291) -> ("Error out"=w286:errorcluster, "TxRx Data"=w287:string[][], "Response Good?"=w288:bool)  [unwired: 4 in]
      }
      frame "Go to Vent Open" {
        n42 = call "EOL CAN_Target Motion.vi"("Rx Arbitration Id"=u32 402522244, "Error in"=w302, "All Motions"=All_Motions."Glass Vent Open", "Read Session in"=w300, "Write Session in"=w301) -> ("Error out"=w296:errorcluster, "TxRx Data"=w297:string[][], "Response Good?"=w298:bool)  [unwired: 4 in]
      }
      frame "Rollo Open" {
        n43 = call "EOL CAN_Target Motion.vi"("Rx Arbitration Id"=u32 402522244, "Error in"=w312, "All Motions"=All_Motions."Sunshade Open", "Read Session in"=w310, "Write Session in"=w311) -> ("Error out"=w306:errorcluster, "TxRx Data"=w307:string[][], "Response Good?"=w308:bool)  [unwired: 4 in]
      }
      frame "Rollo Close" {
        n44 = call "EOL CAN_Target Motion.vi"("Rx Arbitration Id"=u32 402522244, "Error in"=w322, "All Motions"=All_Motions."Sunshade Close", "Read Session in"=w320, "Write Session in"=w321) -> ("Error out"=w316:errorcluster, "TxRx Data"=w317:string[][], "Response Good?"=w318:bool)  [unwired: 4 in]
      }
      frame "Write Vehicle Type" {
        n45 = call "EOL CAN_Write Vehicle Type.vi"("Read Session in"=w324, "Write Session in"=w325) -> ("error out"=w328:errorcluster, "Rx Message"=w326:u8[], "Response Good?"=w327:bool, "Array"=w329:string[][])  [unwired: 6 in]
      }
      frame "Write Shop Code" {
        n46 = call "EOL CAN_Write Repair Shop Code.vi"("Read Session in"=w332, "Write Session in"=w333) -> ("error out"=w336:errorcluster, "Rx Message"=w334:u8[], "Response Good?"=w335:bool, "TxRxData"=w337:string[][])  [unwired: 6 in]
      }
      frame "Download CAL" {
        n47 = call "EOL CAN_Download CAL.vi"("DSC Write Session in"=w358, "Tester"=w344, "Download CAL Time"=w343, "Read Session in"=w357, "Parttype ref"=w340, "Glass?"=TRUE, "ODX File Path"=w342, "Download CAL Progress"=w341) -> ("Response Good?"=w347:bool, "TxRx Data"=w355:string[][], "Error String Out"=→"Error String Out":string, "fail"=w348:bool)  [unwired: 4 in]
        n48 = Not(x=w348) -> (.not. x?=w346:bool)
        n49 = Select(t=Diagnostic_Message."Read SW" ("Enum"), s=w339, f=Diagnostic_Message."Finish Flash" ("Enum")) -> (s? t:f=w351:T2)
        n50 = And(x=w347, y=w346) -> (x .and. y?=→"pass?":bool)
        n51 = Select(t=w351, s=w347, f=Diagnostic_Message."Finish Flash") -> (s? t:f=w350:T2)
      }
      frame "Download FBL" {
        n52 = call "EOL CAN_Download FBL.vi"("DSC Write Session in"=w380, "Tester"=w367, "Download CAL Time"=w366, "Read Session in"=w379, "Parttype ref"=w363, "Glass?"=TRUE, "ODX File Path"=w365, "Download CAL Progress"=w364) -> ("Response Good?"=w361:bool, "TxRx Data"=w377:string[][], "Error String Out"=→"Error String Out 2":string, "fail"=w370:bool)  [unwired: 4 in]
        n53 = Not(x=w370) -> (.not. x?=w369:bool)
        n54 = Select(t=Diagnostic_Message."Read SW" ("Enum"), s=w362, f=Diagnostic_Message."Finish Flash" ("Enum")) -> (s? t:f=w373:T2)
        n55 = And(x=w361, y=w369) -> (x .and. y?=→"pass?_FBL":bool)
        n56 = Select(t=w373, s=w361, f=Diagnostic_Message."Finish Flash") -> (s? t:f=w372:T2)
      }
      frame "Read Vehicle Type" {
        n57 = call "EOL CAN_Get Vehicle type.vi"("Rx Arbitration Id"=u32 402522244, "error in (no error)"=w394, "Tx Arbitration Id"=u32 402391172, "Read Session in"=w393, "Write Session in"=w392) -> ("error out"=w387:errorcluster, "Vehicle Type"=w384:string, "Response Good?"=w388:bool, "TxRx Data"=w389:string[][])  [unwired: 3 in]
        "Vehicle Type" <- w384
        n58 = Bundle By Name(cluster=w386, "Vehicle Type"=w384) -> (w385:T1)
      }
      frame "Clear DTC" {
        n59 = call "EOL CAN_Clear_DTC's.vi"("Error in"=w402, "Read Session in"=w400, "Write Session in"=w401) -> ("Error out"=w399:errorcluster, "TxRx Data"=w397:string[][], "Response Good?"=w398:bool)  [unwired: 6 in]
      }
      frame "Check Teach DTC" {
        n60 = stacked-sequence {
          tunnel: w412 -> [w420 w428]
          tunnel: w411 -> [w419 w427]
          tunnel: [w417 _] -> w408
          tunnel: w410 -> [w418 w426]
          tunnel: [w416 _] -> w406
          tunnel: [_ w425] -> w405
          tunnel: [_ w424] -> w407
          frame #0 {
            n61 = call-poly <vilib>:"XNET Write.vi"("session in"=w420, "data"=T3[] [{"timestamp"=timestamp(0 s since 1904-01-01), "payload"=[2, 16, 79, 85, 85, 85, 85, 85], "identifier"=402391172, "type"=0, "extended?"=TRUE, "echo?"=FALSE}] ("Frame to Send 2"), "error in (no error)"=w419) -> ("error out"=w414:errorcluster)  [unwired: 11 in, 1 out]
            n62 = call "Time Delay22"("error in (no error)"=w414, "Delay Time (s)"=0.05) -> ("error out"=w413:errorcluster)  [unwired: 9 in]
            n63 = call-poly <vilib>:"XNET Read.vi"("session in"=w418, "error in (no error)"=w413) -> ("data"=w416:T3[], "error out"=w417:errorcluster)  [unwired: 10 in, 2 out]
          }
          frame #1 {
            n64 = call-poly <vilib>:"XNET Write.vi"("session in"=w428, "data"=T3[] [{"timestamp"=timestamp(0 s since 1904-01-01), "payload"=[3, 34, 241, 134, 85, 85, 85, 85], "identifier"=402391172, "type"=0, "extended?"=TRUE, "echo?"=FALSE}] ("Frame to Send 2"), "error in (no error)"=w427) -> ("error out"=w423:errorcluster)  [unwired: 11 in, 1 out]
            n65 = call-poly <vilib>:"XNET Read.vi"("session in"=w426, "error in (no error)"=w423) -> ("data"=w425:T3[], "error out"=w424:errorcluster)  [unwired: 10 in, 2 out]
          }
        }
        n66 = Build Array (concatenate)(w406, w405) -> ()  [unwired: 1 out]
        n67 = Merge Errors(w408, w407) -> (w409:errorcluster)
      }
      frame "Finish Flash" {
      }
      frame "Delete RP RF" {
        n68 = call "Time Delay"("error in (no error)"=w434, "Delay Time (s)"=2.5) -> ("error out"=w433:errorcluster)  [unwired: 9 in]
        n69 = call "EOL CAN_Delete RP RF.vi"("error in (no error)"=w433, "Read Session in"=w439, "Write Session in"=w440) -> ("error out"=w436:errorcluster, "Response Good?"=w437:bool, "TxRx Data"=w438:string[][])  [unwired: 6 in]
      }
    }
    "error out" <- w28
    "TxRx Data" <- w24
    "Response Good?" <- w15
    "Rx Message" <- w20
    n70 = Not(x=w15) -> (.not. x?=w14:bool)
    n71 = Equal?(x=w16, y=Diagnostic_Message."Finish Flash" ("Enum")) -> (x = y?=w17:bool)
    n72 = Or(x=w14, y=w17) -> (x .or. y?=w19:bool)
  }
  "ECU Info" <- w3
